vi "External Clock to System Clock.vi"(8 "error in (no error)":errorcluster, 9 "ClockID":u8, 10 "External Time":i64, 11 "CIFCorePlugin in":refnum<class "CIFCorePlugin.lvclass">) -> (0 "error out":errorcluster, 1 "Last Reset Time":i64, 2 "System Time":i64, 3 "CIFCorePlugin out":refnum<class "CIFCorePlugin.lvclass">)   [LabVIEW 2021, in "CIFCorePlugin.lvclass"]
uses:
  CIFCorePlugin.lvclass
  CIFCorePlugin.lvclass/CIFCorePlugin.ctl
  <vilib>/CIF Foundation/CIF Utilities/Time/SubVIs/Add Error.vi
  <vilib>/CIF Foundation/CIF Utilities/Errors/Append Error Location.vi
  <vilib>/CIF Foundation/CIF Utilities/Time/Time_CIF_U.lvlib
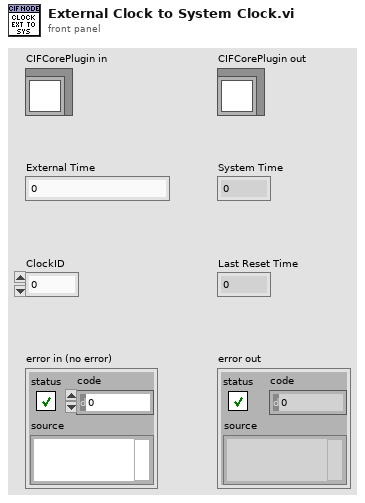
[diagram p1: front panel]
types:
  T1 = typedef "Time_CIF_U.lvlib/Clock Conversion Map.ctl" = map{u8, cluster{"Last Reset":i64, "Offset Pair":T2, "Slope":dbl, "1/Slope":dbl}}
  T2 = typedef "Time_CIF_U.lvlib/Timestamp Pair.ctl" = cluster{"System Time":i64, "External Time":i64}
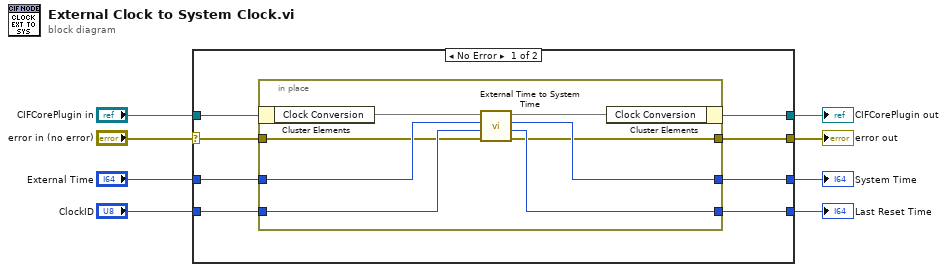
[diagram p0: block diagram]
diagram:
  n1 = case shown="No Error" "error in (no error)" {
    selector: "error in (no error)" -> [w16 w27]
    tunnel: [w15 w27] -> w7
    tunnel: [w14 w26] -> w5
    tunnel: "CIFCorePlugin in" -> [w10 w26]
    tunnel: [w13 w25] -> w4
    tunnel: "External Time" -> [w12 w25]
    tunnel: "ClockID" -> [w11 _]
    tunnel: [w9 _] -> w1
    frame No Error {
      n2 = in-place {
        in-place-border: w16 -> [w18]
        in-place-border: [w17] -> w15
        in-place-border: [w20] -> w13
        in-place-border: w12 -> [w22]
        in-place-border: w11 -> [w21]
        in-place-border: [w19] -> w9
        n3 = in-place-cluster #1(w10) -> ("Clock Conversion"=w24:T1)
        n4 = call <vilib>:"External Time to System Time.vi"("error in (no error)"=w18, "ClockID"=w21, "External Time"=w22, "Clock Convert Map in"=w24) -> ("error out"=w17:errorcluster, "Last Reset Time"=w19:i64, "System Time"=w20:i64, "Clock Convert Map out"=w23:T1)  [unwired: 4 in]
        n5 = in-place-cluster #1("Clock Conversion"=w23) -> (w14:refnum<class "CIFCorePlugin.lvclass">)
      }
    }
    frame Error {
    }
  }
  "error out" <- w7
  "CIFCorePlugin out" <- w5
  "System Time" <- w4
  "Last Reset Time" <- w1
